vi "浮动通知.vi"(10 "通知时间(S)":dbl=3.0, 11 "通知内容":string) -> ()   [LabVIEW 2020]
panel:
  in  "背景颜色":u32(colorbox)
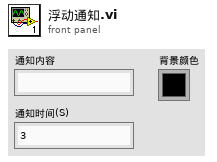
[diagram p1: front panel]
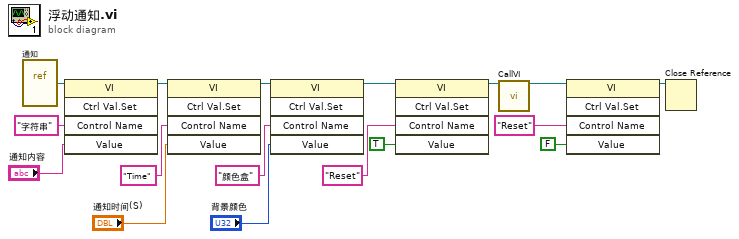
[diagram p0: block diagram]
diagram:
  n1 = vi-ref "通知.vi"() -> (w17:refnum<vi>)
  n2 = invoke class="VI" method="Ctrl Val.Set"(reference=w17, "Control Name"="字符串" ("控件名"), "Value"="通知内容") -> (reference out=w14:refnum<vi>)  [unwired: 2 in, 4 out]
  n3 = invoke class="VI" method="Ctrl Val.Set"(reference=w14, "Control Name"="Time" ("控件名"), "Value"="通知时间(S)") -> (reference out=w4:refnum<vi>)  [unwired: 2 in, 4 out]
  n4 = invoke class="VI" method="Ctrl Val.Set"(reference=w4, "Control Name"="颜色盒" ("控件名"), "Value"="背景颜色") -> (reference out=w3:refnum<vi>)  [unwired: 2 in, 4 out]
  n5 = invoke class="VI" method="Ctrl Val.Set"(reference=w3, "Control Name"="Reset" ("控件名"), "Value"=TRUE) -> (reference out=w6:refnum<vi>)  [unwired: 2 in, 4 out]
  n6 = call "CallVI.vi"("VI引用"=w6) -> ("VI引用输出"=w5:refnum<vi>)  [unwired: 12 in, 2 out]
  n7 = invoke class="VI" method="Ctrl Val.Set"(reference=w5, "Control Name"="Reset" ("控件名"), "Value"=FALSE) -> (reference out=w7:refnum<vi>)  [unwired: 2 in, 4 out]
  n8 = Close Reference(reference=w7) -> ()  [unwired: 1 in, 1 out]
